vi "Do.vi"(8 "error in (no error)":errorcluster, 10 "Actor in":refnum<class "Actor.lvclass">, 11 "Configure Sparse Marker [SM] Msg":refnum<class "Configure Sparse Marker [SM] Msg.lvclass">) -> (0 "error out":errorcluster, 2 "Actor out":refnum<class "Actor.lvclass">)   [LabVIEW 2016, in "CS++Fgen.lvlib" / "Configure Sparse Marker [SM] Msg.lvclass"]
doc: "This VI delivers the message to the actor by calling the appropriate method(s) on the actor."
uses:
  Configure Sparse Marker [SM] Msg.lvclass
  <vilib>/ActorFramework/Actor/Actor.lvclass
  C:/User/Brand/LVP/CSPP-Dev/Packages/CSPP_Core/Actors/CS++PVMonitor Messages/CS++PVUpdate Msg/CS++PVUpdate Msg.lvclass
  CS++Fgen/CS++Fgen.lvclass
  C:/Program Files (x86)/National Instruments/LabVIEW 2016/vi.lib/ActorFramework/Actor/Actor.lvclass
  CSPP_Core/Actors/CS++PVMonitor Messages/CS++PVUpdate Msg/CS++PVUpdate Msg.lvclass/CS++PVUpdate Msg.ctl
  CSPP_Core/Classes/CS++ProcessVariables/ProcessVariable/PV.lvclass/PV.ctl
  Configure Sparse Marker [SM] Msg.lvclass/Configure Sparse Marker [SM] Msg.ctl
  CSPP_Core/Classes/CS++ProcessVariables/ProcessVariable/PV.lvclass
  CSPP_Core/Actors/CS++PVMonitor Messages/CS++PVUpdate Msg/CS++PVUpdate Msg.lvclass
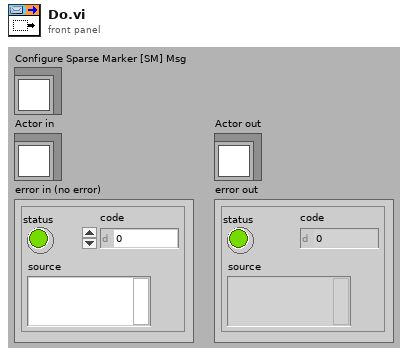
[diagram p1: front panel]
types:
  T1 = cluster{"Marker Name (\"\")":string, "Waveform Handle":i32, "Number Indexes":i64, "Destination Terminal (None)":string, "Indexes Array":i64[]}
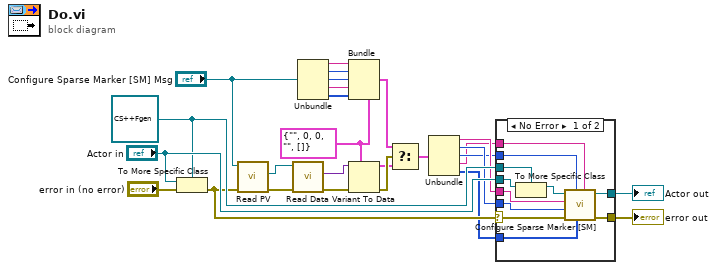
[diagram p0: block diagram]
diagram:
  w18 = T1 {"Marker Name (\"\")"="", "Waveform Handle"=0, "Number Indexes"=0, "Destination Terminal (None)"="", "Indexes Array"=[]} ("Type")
  w22 = refnum<class "CS++Fgen.lvclass"> refnum ("Actor in")
  n1 = To More Specific Class(target class=w22, reference="Actor in", error in="error in (no error)") -> (error out=w11:errorcluster)  [unwired: 1 out]
  n2 = call "Read PV.vi"("error in (no error)"=w11, "CS++PVUpdate Msg in"="Configure Sparse Marker [SM] Msg") -> ("error out"=w21:errorcluster, "PV"=w17:refnum<class "PV.lvclass">)  [unwired: 7 in, 1 out]
  n3 = call "Read Data.vi"("error in (no error)"=w21, "PV in"=w17) -> ("error out"=w15:errorcluster, "Data"=w16:variant)  [unwired: 7 in, 1 out]
  n4 = Unbundle ("Pre-Unbundler")("Configure Sparse Marker [SM] Msg") -> (w5:string, w4:i32, w3:i64, w2:string, w1:i64[])
  n5 = Bundle ("Pre-Bundler")(cluster=w18, "Marker Name (\"\")"=w5, "Waveform Handle"=w4, "Number Indexes"=w3, "Destination Terminal (None)"=w2, "Indexes Array"=w1) -> (w19:T1)
  n6 = Variant To Data(error in=w15, type=w18, Variant=w16) -> (data=w13:T1, error out=w20:errorcluster)
  n7 = Select ("MainSelect")(t=w19, s=w20, f=w13) -> (s? t:f=w14:T1)
  n8 = Unbundle ("Main-Unbundler")(w14) -> ("Marker Name (\"\")"=w10:string, "Waveform Handle"=w9:i32, "Number Indexes"=w8:i64, "Destination Terminal (None)"=w7:string, "Indexes Array"=w6:i64[])
  n9 = case shown="No Error" w11 {
    selector: w11 -> [w35 w39]
    tunnel: [w37 w39] -> w25
    tunnel: [w36 w38] -> w24
    tunnel: "Actor in" -> [w34 w38]
    tunnel: w22 -> [w33 _]
    tunnel: w10 -> [w31 _]
    tunnel: w9 -> [w30 _]
    tunnel: w8 -> [w29 _]
    tunnel: w7 -> [w28 _]
    tunnel: w6 -> [w27 _]
    frame No Error {
      n10 = To More Specific Class(target class=w33, reference=w34) -> (specific class reference=w32:refnum<class "CS++Fgen.lvclass">)  [unwired: 1 in, 1 out]
      n11 = call "Configure Sparse Marker [SM].vi"("Destination Terminal (None)"=w28, "Indexes Array"=w27, "Number Indexes"=w29, "error in (no error)"=w35, "Waveform Handle"=w30, "Marker Name (\"\")"=w31, "CS++Fgen in"=w32) -> ("error out"=w37:errorcluster, "CS++Fgen out"=w36:refnum<class "CS++Fgen.lvclass">)  [unwired: 3 in]
    }
    frame Error {
    }
  }
  "error out" <- w25
  "Actor out" <- w24
